vi "Enable All Defined Programs.vi"() -> ()   [LabVIEW 2010]
uses:
  Drivers/Telemetry/Typedef Command List.ctl
panel:
  out "Affected Programs":string
  out "error out":errorcluster
  in  "error in (no error)":errorcluster
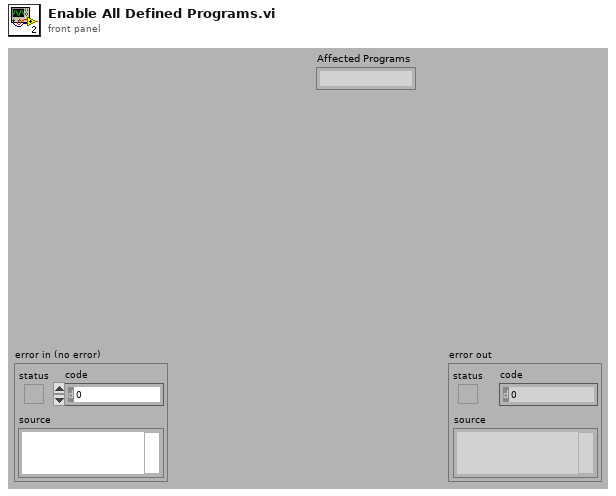
[diagram p1: front panel]
types:
  T1 = enum16{"Open Session", "Close Session", "Downlink Only", "Uplink Only", "Transceive (DN -> UP)"}
  T2 = typedef "Typedef Command List.ctl" = enum16{"Get xPG Status", "xPG Stimulation", "Select Program", "Increment Program Amplitude", "Decrement Program Amplitude", "Get PoP Constants", "Get PPC Constants", "Get Program Names", "Set Pulse Amplitude", "Increment Pulse Amplitude", "Decrement Pulse Amplitude", "Get Pulse Widths", "Set Pulse Widths", "Increment Pulse Width", "Decrement Pulse Width", "Get Program Frequency", "Set Program Frequency", "Increment Program Frequency", "Decrement Program Frequency", "Inject Event", "Charging Control", "Get xPG Identity", "Set xPG Identity", "Restore Program Defaults", "Get Program Definition", "Set Program Definition", "Get Program Constants", "Set Program Constants", "Get Configurable Device Parameters", "Set Configurable Device Parameters", "Get Pulse Constants", "Set Pulse Constants", "Get Lead Limits", "Set Lead Limits", "Get Channel Calibrations", "Set Channel Calibrations", "<reserved 2>", "<reserved 3>", "<reserved 4>", "<reserved 5>", "<reserved 6>", "<reserved 7>", "Get Stim Asic HV Calibrations", "Set Stim Asic HV Calibrations", "<reserved 8>", "<reserved 9>", "Get CP Data", "Set CP Data", "Clear Log", "Read Log", "Append Log", "Get Patient Program Runtime", "Set Patient Program Runtime", "Impedance Measurement", "Enter Storage Mode", "Echo Short", "Echo Long", "Get General Calibration", "Set General Calibration", "Get Trim List", "Set Trim List", "Get Counter", "Set Counter", "Get Test Stimulation", "Set Test Stimulation", "Get Titration Stimulation", "Set Titration Stimulation", "Get Ramp Time", "Set Ramp Time", "Get VBAT", "Set Software Description Block", "Get Software Description Block", "Write Memory", "Read Memory", "Reset xPG", "Erase Flash Block", "Write Vectors", "Read Vectors", "Diagnostic Data", "Set Background Impedance", "Get Background Impedence ", "Undefined"}
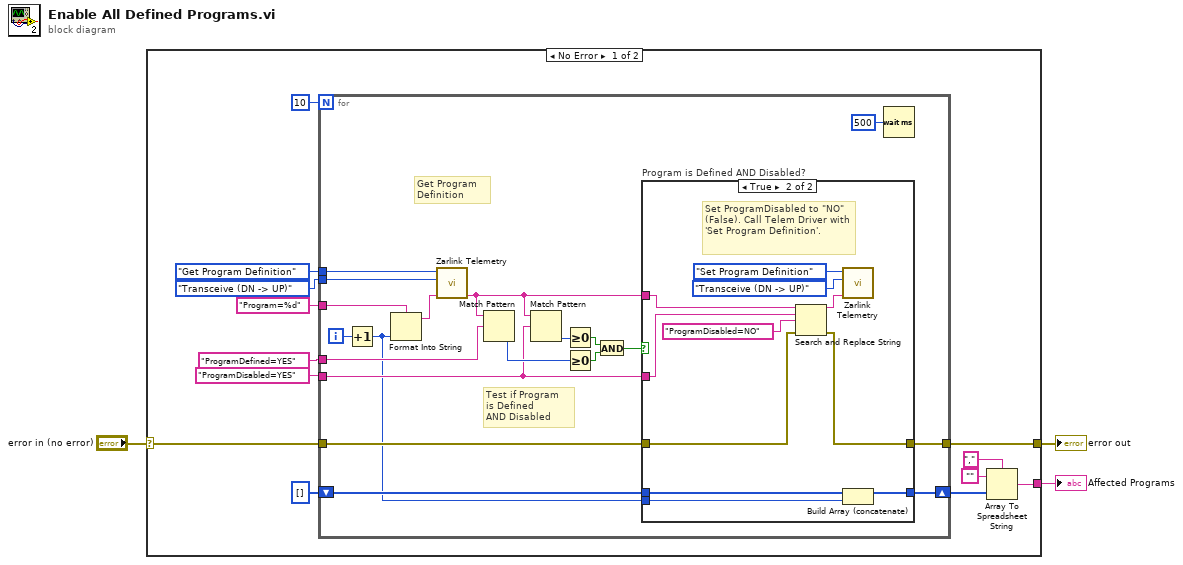
[diagram p0: block diagram]
diagram:
  n1 = case shown="No Error" "error in (no error)" {
    selector: "error in (no error)" -> [w11 w49]
    tunnel: [w10 w49] -> w2
    tunnel: [w4 _] -> w1
    frame No Error {
      n2 = for {
        N: 10 -> [_]
        tunnel: Typedef_Command_List."Get Program Definition" ("Command") -> [w35]
        tunnel: T1."Transceive (DN -> UP)" ("Function") -> [w34]
        tunnel: "Program=%d" -> [w32]
        tunnel: "ProgramDefined=YES" ("regular expression") -> [w30]
        tunnel: "ProgramDisabled=YES" ("regular expression") -> [w23]
        tunnel: w11 -> [w22]
        tunnel: [w21] -> w10
        shift-right: [w20] -> w7
        shift-left: i32[] [] -> [w19]
        i -> [w31]
        # "Test if Program\nis Defined\nAND Disabled"
        # "Get Program\nDefinition"
        n3 = Increment(x=w31) -> (x+1=w18:i32)
        n4 = Format Into String(format string=w32, w18) -> (resulting string=w33:string)  [unwired: 2 in, 1 out]
        n5 = call "Zarlink Telemetry.vi"("Parameters"=w33, "Function"=w34, "Command"=w35) -> ("Data"=w24:string)  [unwired: 3 in, 5 out]
        n6 = Match Pattern(string=w24, regular expression=w30) -> (offset past match=w29:i32)  [unwired: 1 in, 3 out]
        n7 = Match Pattern(string=w24, regular expression=w23) -> (offset past match=w28:i32)  [unwired: 1 in, 3 out]
        n8 = Greater Or Equal To 0?(x=w28) -> (x >= 0?=w26:bool)
        n9 = Greater Or Equal To 0?(x=w29) -> (x >= 0?=w27:bool)
        n10 = And(x=w26, y=w27) -> (x .and. y?=w25:bool)
        n11 = case "Program is Defined AND Disabled?" shown="True" w25 {
          tunnel: w24 -> [_ w48]
          tunnel: w23 -> [_ w47]
          tunnel: w22 -> [w37 w45]
          tunnel: [w37 w44] -> w21
          tunnel: w18 -> [_ w40]
          tunnel: [w36 w39] -> w20
          tunnel: w19 -> [w36 w38]
          frame False {
          }
          frame True {
            # "Set ProgramDisabled to \"NO\" (False). Call Telem Driver with 'Set Program Definition'."
            n12 = Search and Replace String(input string=w48, search string=w47, replace string="ProgramDisabled=NO" ("regular expression"), error in=w45) -> (result string=w43:string, error out=w44:errorcluster)  [unwired: 4 in, 2 out]
            n13 = call "Zarlink Telemetry.vi"("Parameters"=w43, "Function"=T1."Transceive (DN -> UP)", "Command"=Typedef_Command_List."Set Program Definition") -> ()  [unwired: 3 in, 6 out]
            n14 = Build Array (concatenate)(w38, w40) -> (w39:i32[])
          }
        }
        n15 = Wait (ms)(milliseconds to wait=u32 500) -> ()  [unwired: 1 out]
      }
      n16 = Array To Spreadsheet String(delimiter (Tab)=",", array=w7, 3:"") -> (spreadsheet string=w4:string)
    }
    frame Error {
    }
  }
  "error out" <- w2
  "Affected Programs" <- w1
